vi "PPMSDR Monitor and Control.vi"(8 "Refresh Rate":dbl=1.346, 11 "IP Address":string="130.49.180.18") -> ()   [LabVIEW 2013]
doc: "This VI monitors the PPMS temperature and magnetic field using QD Labview interface. These values are continuously updated to a global variable."
uses:
  user/michelle/QDServer/QDServGlobal.vi
panel:
  in  "Stop Button":bool
  out "Temperature":dbl=300.0041
  out "Field":dbl=-0.014
  out "Temperature\nStatus":i32(ring)=1 items=["TemperatureUnknown"=0, "Stable"=1, "Tracking"=2, "Near"=5, "Chasing"=6, "Filling"=7, "Standby"=10, "Disabled"=13, "ImpedanceNotFunction"=14, "TempFailure"=15]
  out "Field\nStatus":i32(ring)=1 items=["MagnetUnknown"=0, "StablePersistent"=1, "WarmingSwitch"=2, "CoolingSwitch"=3, "StableDriven"=4, "Iterating"=5, "Charging"=6, "Discharging"=7, "CurrentError"=8, "MagnetFailure"=15]
  out "Rate (K/min)":dbl=20.0
  out "Target Temp":dbl=300.0
  out "Mode":enum16{"Persistent", "Driven"}(ring)
  out "Rate (Oe/s)":dbl=100.0
  out "Target Field":dbl
  out "Set Temp?":bool
  out "Set Field?":bool
  in  "Temp Approach":enum16{"FastSettle", "NoOvershoot"}(ring)
  # "PPMS-DR Server"
  # "1. Open the QD server \n    on PPMS computer\n\n2. Get the IP address \n     and run."
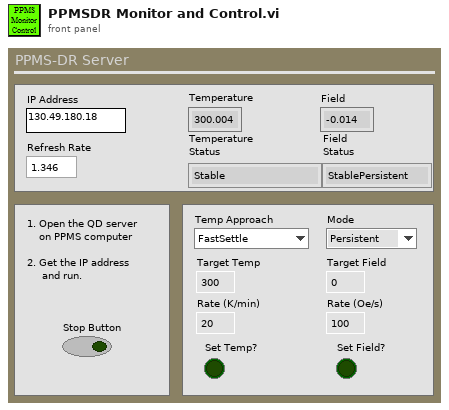
[diagram p1: front panel]
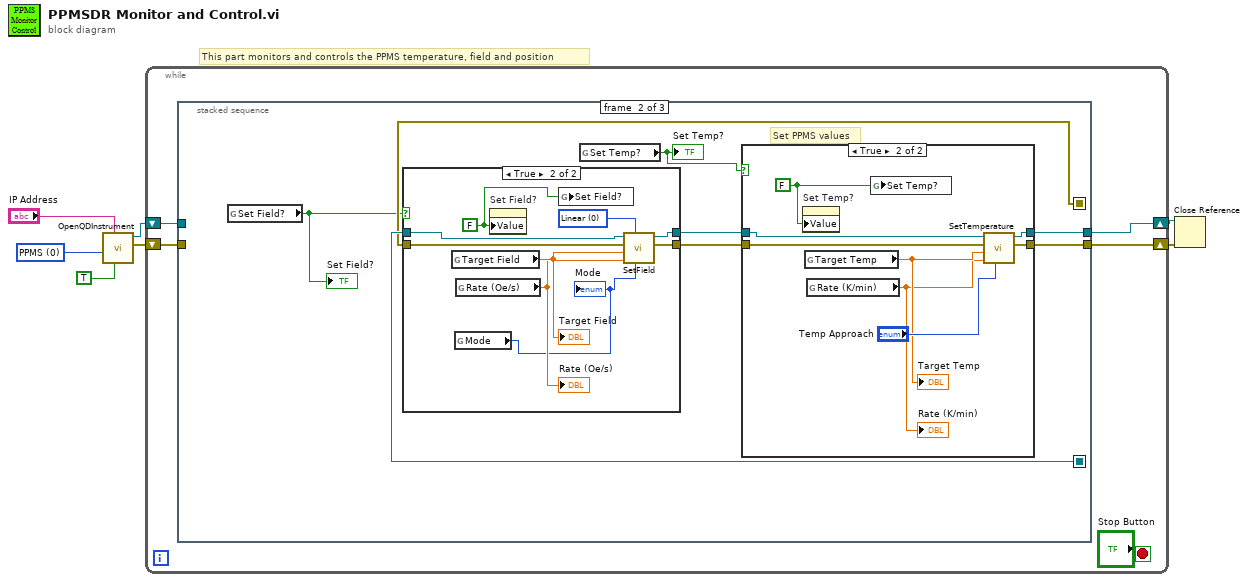
[diagram p0: block diagram]
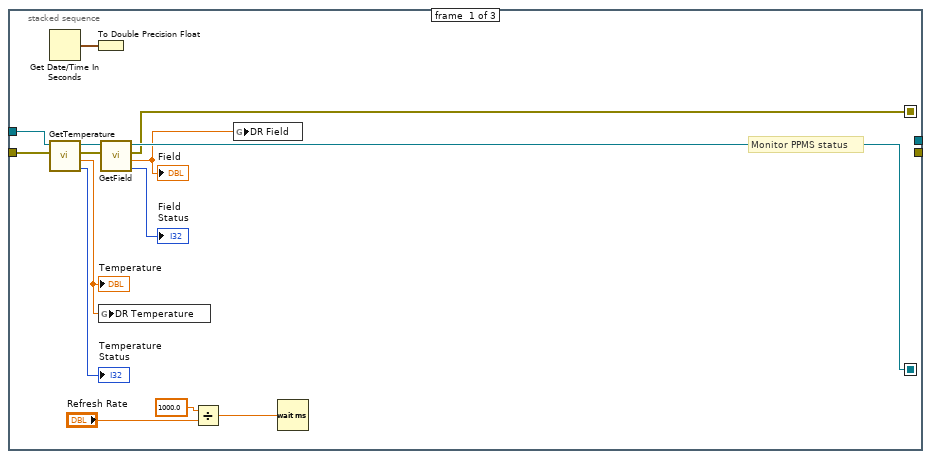
[diagram p2: hidden frame]
diagram:
  w5 = 0 items=["PPMS", "VersaLab", "DynaCool", "SVSM"] ("Instrument\nType")
  # "This part monitors and controls the PPMS temperature, field and position"
  n1 = call "OpenQDInstrument.vi"("Remote"=TRUE, "IP Address"="IP Address", "Instrument Type"=w5) -> ("error out"=w3:errorcluster, "Instrument Ref"=w4:refnum<k24>)  [unwired: 5 in]
  n2 = while {
    shift-right: [w10] -> w2
    shift-left: w4 -> [w12]
    shift-right: [w9] -> w1
    shift-left: w3 -> [w11]
    stop <- "Stop Button" stop-if-true
    n3 = stacked-sequence {
      seq-local: [w17 _ _] -> [_ w34 _]
      seq-local: [w16 _ _] -> [_ w33 _]
      tunnel: w12 -> [w26 _ _]
      tunnel: w11 -> [w25 _ _]
      tunnel: [_ w30 _] -> w10
      tunnel: [_ w29 _] -> w9
      frame #0 {
        # "Monitor PPMS status"
        n4 = Get Date/Time In Seconds() -> (seconds since 1Jan1904=w23:timestamp)
        n5 = call "GetTemperature.vi"("error in (no error)"=w25, "Instrument Ref In"=w26) -> ("Temperature\nStatus"=→"Temperature\nStatus":i32, "Temperature"=w14:dbl, "error out"=w22:errorcluster, "Instrument Ref Out"=w21:refnum<k24>)  [unwired: 3 in, 1 out]
        "Temperature" <- w14
        n6 = To Double Precision Float(number=w23) -> ()  [unwired: 1 out]
        n7 = global write "QDServGlobal.vi" "DR Temperature"(w14) -> ()
        n8 = call "GetField.vi"("error in (no error)"=w22, "Instrument Ref In"=w21) -> ("Field\nStatus"=→"Field\nStatus":i32, "Field"=w15:dbl, "error out"=w16:errorcluster, "Instrument Ref Out"=w17:refnum<k24>)  [unwired: 3 in, 1 out]
        "Field" <- w15
        n9 = Divide(x=1000.0 ("milliseconds to wait"), y="Refresh Rate") -> (x/y=w18:dbl)
        n10 = global write "QDServGlobal.vi" "DR Field"(w15) -> ()
        n11 = Wait (ms)(milliseconds to wait=w18) -> ()  [unwired: 1 out]
      }
      frame #1 {
        # "Set PPMS values"
        n12 = global read "QDServGlobal.vi" "Set Field?"() -> (w28:bool)
        "Set Field?" <- w28
        n13 = case shown="True" w28 {
          tunnel: w34 -> [w46 w54]
          tunnel: w33 -> [w45 w53]
          tunnel: [w46 w52] -> w32
          tunnel: [w45 w51] -> w31
          frame False {
          }
          frame True {
            w50 = FALSE ("Set Field?")
            w55 = 0 items=["Linear", "NoOvershoot", "Oscillate"] ("Approach")
            n14 = global read "QDServGlobal.vi" "Target Field"() -> (w49:dbl)
            "Target Field" <- w49
            n15 = global read "QDServGlobal.vi" "Mode"() -> (w47:enum16{"Persistent", "Driven"})
            "Mode" <- w47
            n16 = global read "QDServGlobal.vi" "Rate (Oe/s)"() -> (w48:dbl)
            "Rate (Oe/s)" <- w48
            n17 = property on="Set Field?" class="Bool (strict)"("Value"=w50) -> ()  [unwired: 2 in, 2 out]
            n18 = global write "QDServGlobal.vi" "Set Field?"(w50) -> ()
            n19 = call "SetField.vi"("Mode"=w47, "Approach"=w55, "Rate"=w48, "Field"=w49, "error in (no error)"=w53, "Instrument Ref In"=w54) -> ("error out"=w51:errorcluster, "Instrument Ref Out"=w52:refnum<k24>)  [unwired: 1 in, 1 out]
          }
        }
        n20 = global read "QDServGlobal.vi" "Set Temp?"() -> (w27:bool)
        "Set Temp?" <- w27
        n21 = case shown="True" w27 {
          tunnel: w32 -> [w36 w43]
          tunnel: w31 -> [w35 w42]
          tunnel: [w36 w41] -> w30
          tunnel: [w35 w40] -> w29
          frame False {
          }
          frame True {
            w39 = FALSE ("Set Temp?")
            n22 = property on="Set Temp?" class="Bool (strict)"("Value"=w39) -> ()  [unwired: 2 in, 2 out]
            n23 = global read "QDServGlobal.vi" "Target Temp"() -> (w38:dbl)
            "Target Temp" <- w38
            n24 = global read "QDServGlobal.vi" "Rate (K/min)"() -> (w37:dbl)
            "Rate (K/min)" <- w37
            n25 = global write "QDServGlobal.vi" "Set Temp?"(w39) -> ()
            n26 = call "SetTemperature.vi"("Approach"="Temp Approach", "Rate"=w37, "Temperature"=w38, "error in (no error)"=w42, "Instrument Ref In"=w43) -> ("error out"=w40:errorcluster, "Instrument Ref Out"=w41:refnum<k24>)  [unwired: 2 in, 1 out]
          }
        }
      }
      frame #2 {
      }
    }
  }
  n27 = Close Reference(reference=w2, error in (no error)=w1) -> ()  [unwired: 1 out]
